vi "sub vi - Make Directory.vi"(10 "Path":string="C:\\Documents and Settings\\Peter\\Desktop\\data\\", 11 "date format (0)":enum16{"short", "long", "abbreviated"}(ring)) -> (2 "directory":string, 3 "date string":string)   [LabVIEW 2010]
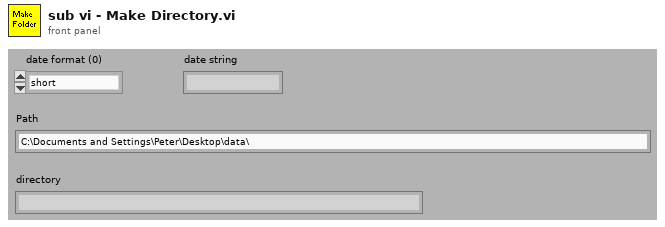
[diagram p1: front panel]
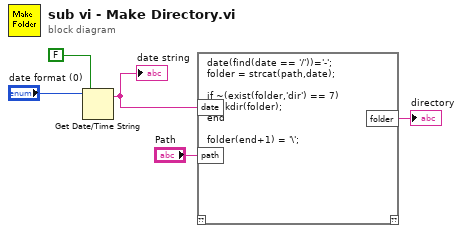
[diagram p0: block diagram]
diagram:
  n1 = Get Date/Time String(date format (0)="date format (0)", want seconds? (F)=FALSE) -> (date string=w3:string)  [unwired: 2 out]
  "date string" <- w3
  n2 = script code="date(find(date == '/'))='-';\nfolder = strcat(path,date);\n\nif ~(exist(folder,'dir') == 7)\n   mkdir(folder);\nend\n\nfolder(end+1) = '\\';"("date"=w3, "path"="Path") -> ("folder"=→"directory":string)  [unwired: 2 out]
